vi "TestStand_Control ( Execution_View_Callback ).vi"(4 "TestStand UI Data":T1, 5 "Event Data":cluster{"exec":refnum<k7>, "reason":i32}, 6 "Control Ref":refnum<k7>, 7 "Event Common Data":T2) -> ()   [LabVIEW 2018, in "TestStand_Control.lvlib"]
uses:
  Module_Controls/TestStand UI Data.ctl
  TestStand_Control.lvlib
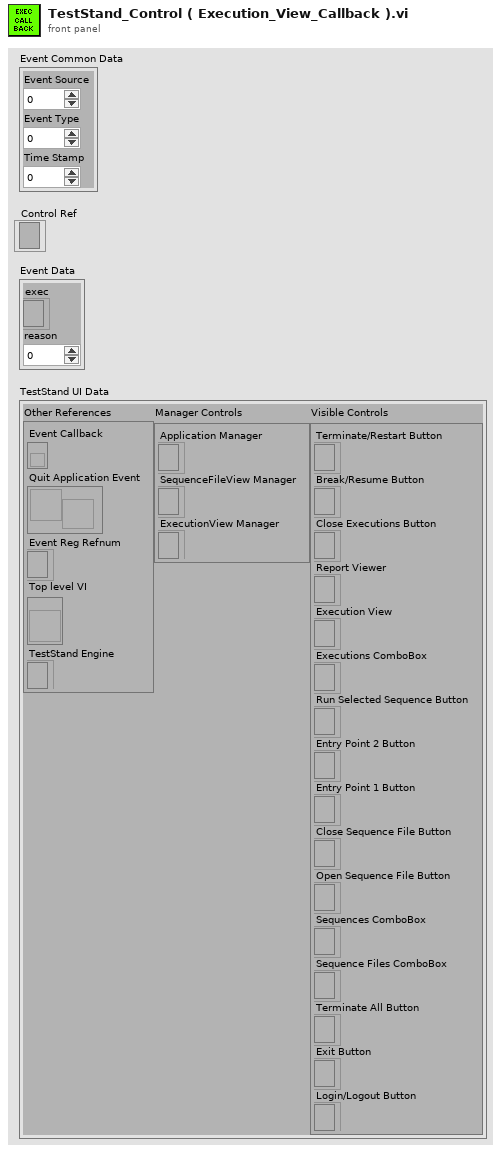
[diagram p1: front panel]
types:
  T1 = typedef "TestStand_Control.lvlib/TestStand UI Data.ctl" = cluster{"Other References":cluster{"Event Callback":refnum<k27>, "Quit Application Event":refnum<user-event>, "Event Reg Refnum":refnum<event-registration>, "Top level VI":refnum<vi>, "TestStand Engine":refnum<k7>}, "Manager Controls":cluster{"Application Manager":refnum<k7>, "SequenceFileView Manager":refnum<k7>, "ExecutionView Manager":refnum<k7>}, "Visible Controls":cluster{"Terminate/Restart Button":refnum<k7>, "Break/Resume Button":refnum<k7>, "Close Executions Button":refnum<k7>, "Report Viewer":refnum<k7>, "Execution View":refnum<k7>, "Executions ComboBox":refnum<k7>, "Run Selected Sequence Button":refnum<k7>, "Entry Point 2 Button":refnum<k7>, "Entry Point 1 Button":refnum<k7>, "Close Sequence File Button":refnum<k7>, "Open Sequence File Button":refnum<k7>, "Sequences ComboBox":refnum<k7>, "Sequence Files ComboBox":refnum<k7>, "Terminate All Button":refnum<k7>, "Exit Button":refnum<k7>, "Login/Logout Button":refnum<k7>}}
  T2 = cluster{"Event Source":i32, "Event Type":u32, "Time Stamp":u32}
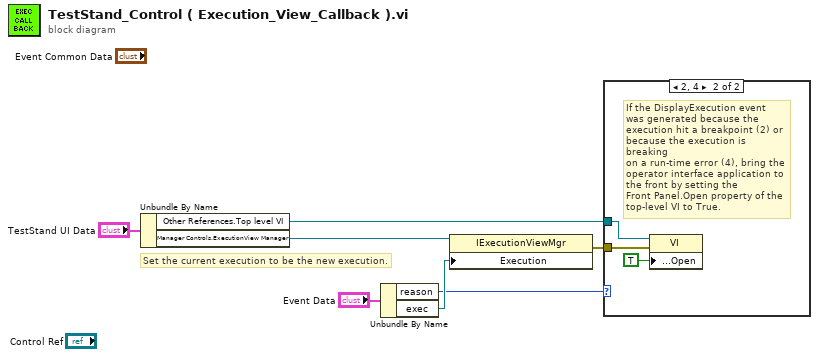
[diagram p0: block diagram]
diagram:
  # "Set the current execution to be the new execution."
  n1 = Unbundle By Name("TestStand UI Data") -> ("Other References.Top level VI"=w1:refnum<vi>, "Manager Controls.ExecutionView Manager"=w5:refnum<k7>)
  n2 = Unbundle By Name("Event Data") -> ("reason"=w2:i32, "exec"=w3:refnum<k7>)
  n3 = property class="IExecutionViewMgr"(reference=w5, "Execution"=w3) -> (error out=w7:errorcluster)  [unwired: 1 in, 1 out]
  n4 = case shown="2, 4" w2 {
    tunnel: w7 -> [_ w10]
    tunnel: w1 -> [_ w8]
    frame Default {
    }
    frame 2, 4 {
      # "If the DisplayExecution event\nwas generated because the\nexecution hit a breakpoint (2) or\nbecause the execution is breaking\non a run-time error (4), bring the\noperator interface application to\nthe front by setting the\nFront Panel.Open property of the\ntop-level VI to True."
      n5 = property class="VI"(reference=w8, error in=w10, "Front Panel Window:Open"=TRUE) -> ()  [unwired: 2 out]
    }
  }
